vi "bats.parser.test.vi"() -> ()   [LabVIEW 2022 SP3]
uses:
  <vilib>/Platform/TimedLoop/XDataNode/timing_clust.ctl
  <vilib>/Platform/TimedLoop/XDataNode/nitl_modes.ctl
  <vilib>/Platform/TimedLoop/XDataNode/wakeup.ctl
  <vilib>/rvi/DataTransferAndStorage/Container/Common/niFpgaContainerGetUniqueNameForEmu.vi
  <vilib>/rvi/DataTransferAndStorage/Container/Common/niFpgaContainerSetEmuInfo.vi
  <vilib>/rvi/eio/common/nirviEmuReportErrorAndStop.vi
  <vilib>/rvi/Emulation/niFpgaSctlEmulationGetInTimedLoop.vi
  <vilib>/rvi/Emulation/niFpgaEmulationReportErrorSimple.vi
  <vilib>/rvi/Emulation/niFpgaGetClockAttributes.vi
  <vilib>/rvi/Emulation/niFpgaCriticalErrorInLSC.vi
  <vilib>/rvi/interface/RandomDataEmulation/nirviRandomDataMultiElementFPGAFIFO.vi
  <instcachedir>/0/nirviRandomDataMultiElementFPGAFIFO_3E9965BA1FAD4E7B8DABA31768A09B1F.lvgen/nirviRandomDataMultiElementFPGAFIFO_3E9965BA1FAD4E7B8DABA31768A09B1F_003.vi
  <vilib>/rvi/interface/RandomDataEmulation/niFpgaRandomDataHandleErrors.vi
  <vilib>/rvi/DataTransferAndStorage/Container/Common/niFpgaContainerExecOnDevCompGetState.vi
  <vilib>/rvi/Emulation/niFpgaEmulationIsFPGAContextNoSignature.vi
  <vilib>/rvi/errors/niFpgaSetErrorForExecOnDevCompSimple.vi
  <vilib>/rvi/FIFO/Fifo_Resource/nirvififoEmulationSetSize.vi
  <vilib>/rvi/FIFO/Fifo_Resource/nirviFifoEmulationQueueMgr.vi
  <instcachedir>/0/nirviFifoEmulationQueueMgr_E5CAEC123FF24DC58D834DCA3CDAA9B5.lvgen/nirviFifoEmulationQueueMgr_E5CAEC123FF24DC58D834DCA3CDAA9B5_009.vi
  <vilib>/rvi/FIFO/Fifo_Resource/nirvififoEmulationDetermineInputValidOut.vi
  <vilib>/rvi/FIFO/Fifo_Resource/nirvififoEmulationCreateLock.vi
  <vilib>/rvi/Emulation/niFpgaProcessEmulError.vi
  <vilib>/rvi/FIFO/Fifo_Resource/nirvififoEmulationObtainLock.vi
  <vilib>/rvi/FIFO/Fifo_Resource/nirvififoEmulationReleaseLock.vi
  <vilib>/rvi/occurrence/nirviWaitOnOccurrenceBase.vi
  <vilib>/rvi/errors/nirviReportUnexpectedCaseInternalError.vi
  <vilib>/rvi/errors/nirviReportUnexpectedCaseInternalError (U32).vi
  <vilib>/Utility/error.llb/Clear Errors.vi
  <instcachedir>/0/nirviFifoEmulationQueueMgr_E5CAEC123FF24DC58D834DCA3CDAA9B5.lvgen/nirviFifoEmulationQueueMgr_E5CAEC123FF24DC58D834DCA3CDAA9B5_026.vi
  <instcachedir>/0/nirviRandomDataMultiElementFPGAFIFO_3E9965BA1FAD4E7B8DABA31768A09B1F.lvgen/nirviRandomDataMultiElementFPGAFIFO_3E9965BA1FAD4E7B8DABA31768A09B1F_001.vi
  <instcachedir>/0/nirviFifoEmulationQueueMgr_E5CAEC123FF24DC58D834DCA3CDAA9B5.lvgen/nirviFifoEmulationQueueMgr_E5CAEC123FF24DC58D834DCA3CDAA9B5_000.vi
  <vilib>/Platform/TimedLoop/XDataNode/XDataNode.xnode
  <vilib>/rvi/LocalResourceManager/LocalResourceManager.xnode
  <vilib>/rvi/DataTransferAndStorage/Container/XNode/niFpgaContainer.xnode
  <vilib>/rvi/interface/RandomDataEmulation/nirviRandomDataFpgaMultiElementTemplate.vi
  <vilib>/rvi/FIFO/Fifo_Resource/niFpgaFifoEmulationRefIn.vi
  <vilib>/rvi/FIFO/Fifo_Resource/nirvififoEmulationRead.vi
  <vilib>/rvi/interface/RandomDataEmulation/nirviRandomDataFpgaReadWriteTemplate.vi
  <vilib>/Platform/TimedLoop/XDataNode/XDNodeRunTimeDep.lvlib
panel:
  in  "reset":bool
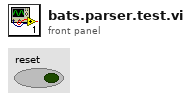
[diagram p1: front panel]
types:
  T1 = typedef "XDNodeRunTimeDep.lvlib/timing_clust.ctl" = cluster{"Expected End [f-1]":u64, "Actual End [f-1]":u64, "Finished Late? [f-1]":bool, "Expected End [i-1]":u64, "Actual End [i-1]":u64, "Finished Late? [i-1]":bool, "Expected Start [i]":u64, "Actual Start [i]":u64, "Expected Start [f]":u64, "Actual Start [f]":u64, "Source Name":string, "Structure Name":string, "Period":i64, "Deadline":i64, "Offset":i64, "Start":i64, "Priority":i32, "Timeout":i32, "Mode":T2, "Wakeup Reason":T3, "Error":errorcluster, "Source Type":string, "Secondary Source Type":string, "Global End Time":u64, "Global Start Time":u64, "Frame Duration":u64, "Iteration Duration":u64, "Assigned CPU":i32, "I/O Scan Engine Mode":u32}
  T2 = typedef "XDNodeRunTimeDep.lvlib/nitl_modes.ctl" = enum32{"No Change", "Process missed periods, maintain original phase", "Discard missed periods, maintain original phase", "Process missed periods, ignore original phase", "Discard missed periods, ignore original phase"}
  T3 = typedef "XDNodeRunTimeDep.lvlib/wakeup.ctl" = enum32{"Normal", "Aborted", "Asynchronous wakeup", "Timing source error", "Timed loop error", "Timeout"}
  T4 = typedef "data.ctl" = cluster{"enabled":bool[], "byte":u8[]}
  T5 = cluster{"type":enum8{"Time", "AddOrder", "OrderExecuted", "OrderExecutedAtPrice", "ReduceSize", "ModifyOrder", "DeleteOrder", "Get.Everything", "Get.All.Orders", "Get.Top"}, "side":u8, "orderId ":u64, "quantity":u32, "symbol":u64, "price":u64, "executed.qty":u32, "canceled.qty":u32, "remaining.qty":u32, "seconds":u64, "nanoseconds":u64, "Add":bool, "Edit":bool, "Remove":bool}
  T6 = enum8{"Time", "AddOrder", "OrderExecuted", "OrderExecutedAtPrice", "ReduceSize", "ModifyOrder", "DeleteOrder", "Get.Everything", "Get.All.Orders", "Get.Top"}
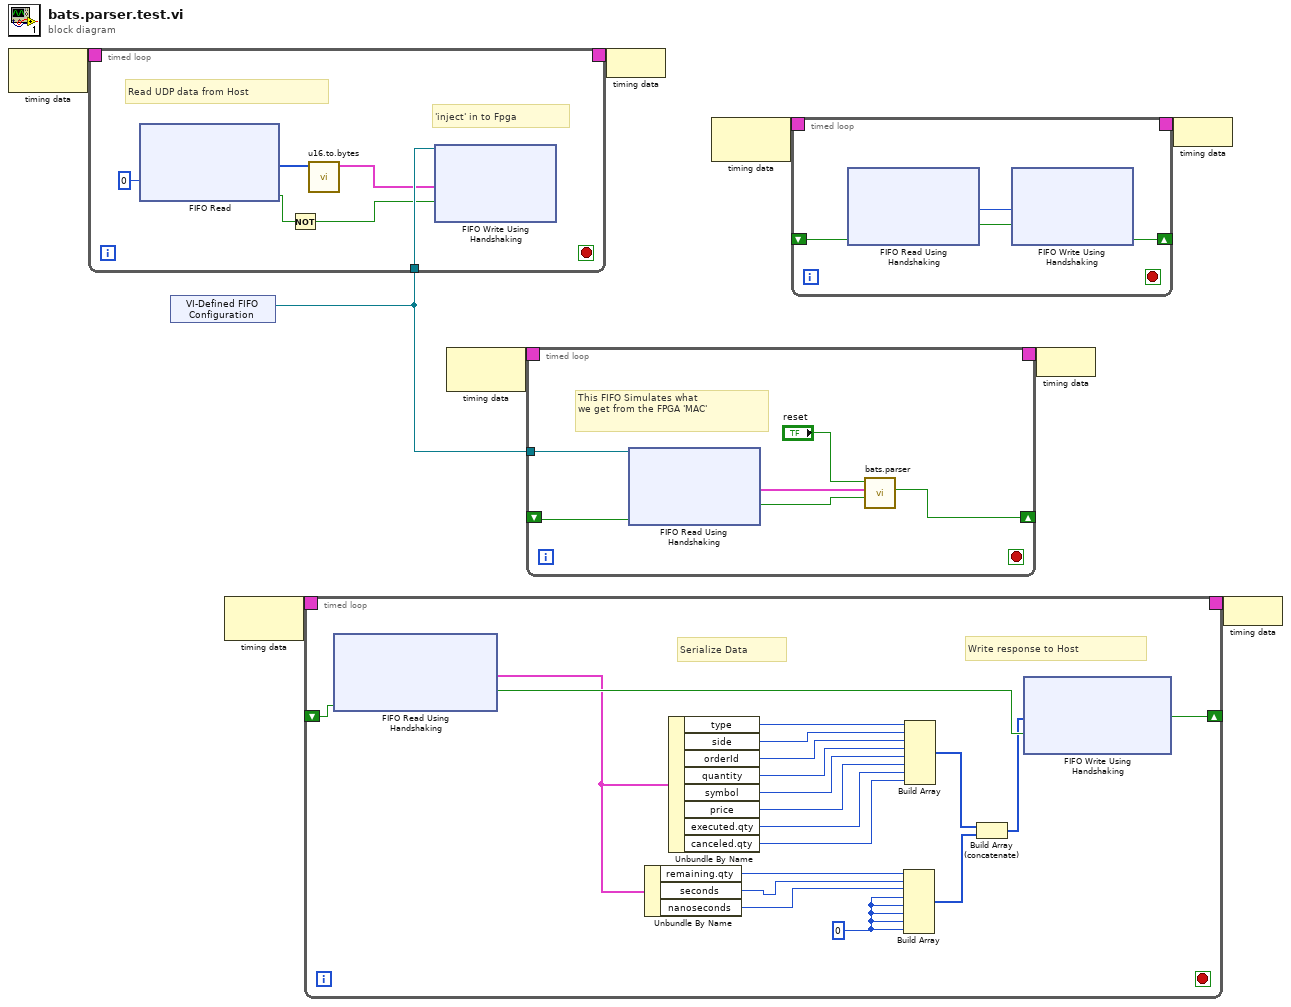
[diagram p0: block diagram]
diagram:
  n1 = node-c288() -> (w9:T1)  [unwired: 1 in]
  n2 = xnode "VI-Defined FIFO Configuration"() -> ("FIFO Out"=w5:refnum<k21>)
  n3 = timed-loop {
    timing: w9 -> [_]
    timing-out: [_] -> w8
    tunnel: w5 -> [w15]
    stop <- _ stop-if-true
    # "'inject' in to Fpga"
    # "Read UDP data from Host"
    n4 = xnode ("FIFO Read")("Timeout"=0) -> ("Element"=w11:u16[], "Timed Out?"=w13:bool)  [unwired: 1 in, 1 out]
    n5 = Not(x=w13) -> (.not. x?=w12:bool)
    n6 = call "u16.to.bytes.vi"("data.u16.in"=w11) -> ("data"=w10:T4)  [unwired: 10 in]
    n7 = xnode ("FIFO Write Using Handshaking")("Element"=w10, "Input Valid"=w12, "FIFO In"=w15) -> ()  [unwired: 2 out]
  }
  n8 = node-c288() -> (w4:T1)  [unwired: 1 in]
  n9 = timed-loop {
    timing: w4 -> [_]
    timing-out: [_] -> w3
    shift-right: [w36] -> _
    shift-left: _ -> [w27]
    stop <- _ stop-if-true
    w20 = u64 0 ("element")
    # "Serialize Data"
    # "Write response to Host"
    n10 = xnode ("FIFO Read Using Handshaking")("Ready for Output"=w27) -> ("Element"=w22:T5, "Output Valid"=w26:bool)  [unwired: 1 in, 1 out]
    n11 = Unbundle By Name(w22) -> ("remaining.qty"=w21:u32, "seconds"=w18:u64, "nanoseconds"=w19:u64)
    n12 = Unbundle By Name(w22) -> ("type"=w35:T6, "side"=w34:u8, "orderId"=w33:u64, "quantity"=w32:u32, "symbol"=w31:u64, "price"=w30:u64, "executed.qty"=w29:u32, "canceled.qty"=w28:u32)
    n13 = Build Array(w21, w18, w19, w20, w20, w20, w20, w20) -> (w23:u64[])
    n14 = Build Array(w35, w34, w33, w32, w31, w30, w29, w28) -> (w25:u64[])
    n15 = Build Array (concatenate)(w25, w23) -> (w24:u64[])
    n16 = xnode ("FIFO Write Using Handshaking")("Element"=w24, "Input Valid"=w26) -> ("Ready for Input"=w36:bool)  [unwired: 1 in, 1 out]
  }
  n17 = node-c288() -> (w7:T1)  [unwired: 1 in]
  n18 = timed-loop {
    timing: w7 -> [_]
    timing-out: [_] -> w6
    tunnel: w5 -> [w44]
    shift-right: [w43] -> _
    shift-left: _ -> [w42]
    stop <- _ stop-if-true
    # "This FIFO Simulates what\nwe get from the FPGA 'MAC'"
    n19 = xnode ("FIFO Read Using Handshaking")("Ready for Output"=w42, "FIFO In"=w44) -> ("Element"=w41:cluster{"enabled":bool[], "byte":u8[]}, "Output Valid"=w39:bool)  [unwired: 1 out]
    n20 = call "bats.parser.vi"("data.valid"=w39, "data"=w41, "reset"="reset") -> ("Ready.for.Udp.Input"=w43:bool)  [unwired: 8 in]
  }
  n21 = node-c288(w8) -> ()
  n22 = node-c288() -> (w2:T1)  [unwired: 1 in]
  n23 = timed-loop {
    timing: w2 -> [_]
    timing-out: [_] -> w1
    shift-right: [w50] -> _
    shift-left: _ -> [w49]
    stop <- _ stop-if-true
    n24 = xnode ("FIFO Read Using Handshaking")("Ready for Output"=w49) -> ("Element"=w47:u64, "Output Valid"=w48:bool)  [unwired: 1 in, 1 out]
    n25 = xnode ("FIFO Write Using Handshaking")("Element"=w47, "Input Valid"=w48) -> ("Ready for Input"=w50:bool)  [unwired: 1 in, 1 out]
  }
  n26 = node-c288(w6) -> ()
  n27 = node-c288(w1) -> ()
  n28 = node-c288(w3) -> ()
